vi "Read Data Buffer Subset.vi"(0 "VISA resource name":refnum<visa-resource-name>, 1 "All Data Elements (False)":bool, 2 "Timeout (30000 milliseconds)":u32=30000, 5 "Previous Buffer Read Location (0)":i32, 7 "Next Buffer Location (0)":i32, 9 "Buffer Size (1000)":i32=1000, 11 "error in (no error)":errorcluster) -> (4 "VISA resource name out":refnum<visa-resource-name>, 6 "Measurement Data":dbl[](array[numeric]), 8 "Timestamp":string[](array[string]), 10 "Channel":string[](array[string]), 14 "Reading Number":string[](array[string]), 15 "error out":errorcluster)   [LabVIEW 2020, in "Keithley 27XX.lvlib"]
doc: "It fetches data from the data buffer given the previous buffer location read, and the next buffer location. This VI alone does not initiate a measurement.\n\nNote:\n(1) This VI can be used with continuous initiation to do continuous reads.\n\n(2) Returning all data elements requires ASCII transfers.\n\n(3) Timestamp, Channel, and Reading Number arrays will be left empty if the All Data Elements control is set to False."
uses:
  <instrlib>/Keithley 27XX/Keithley 27XX.lvlib
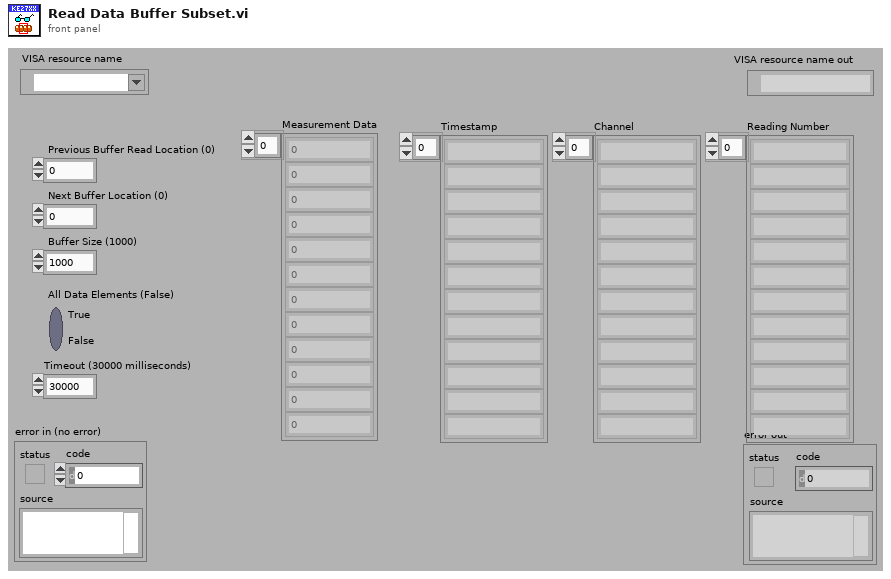
[diagram p1: front panel]
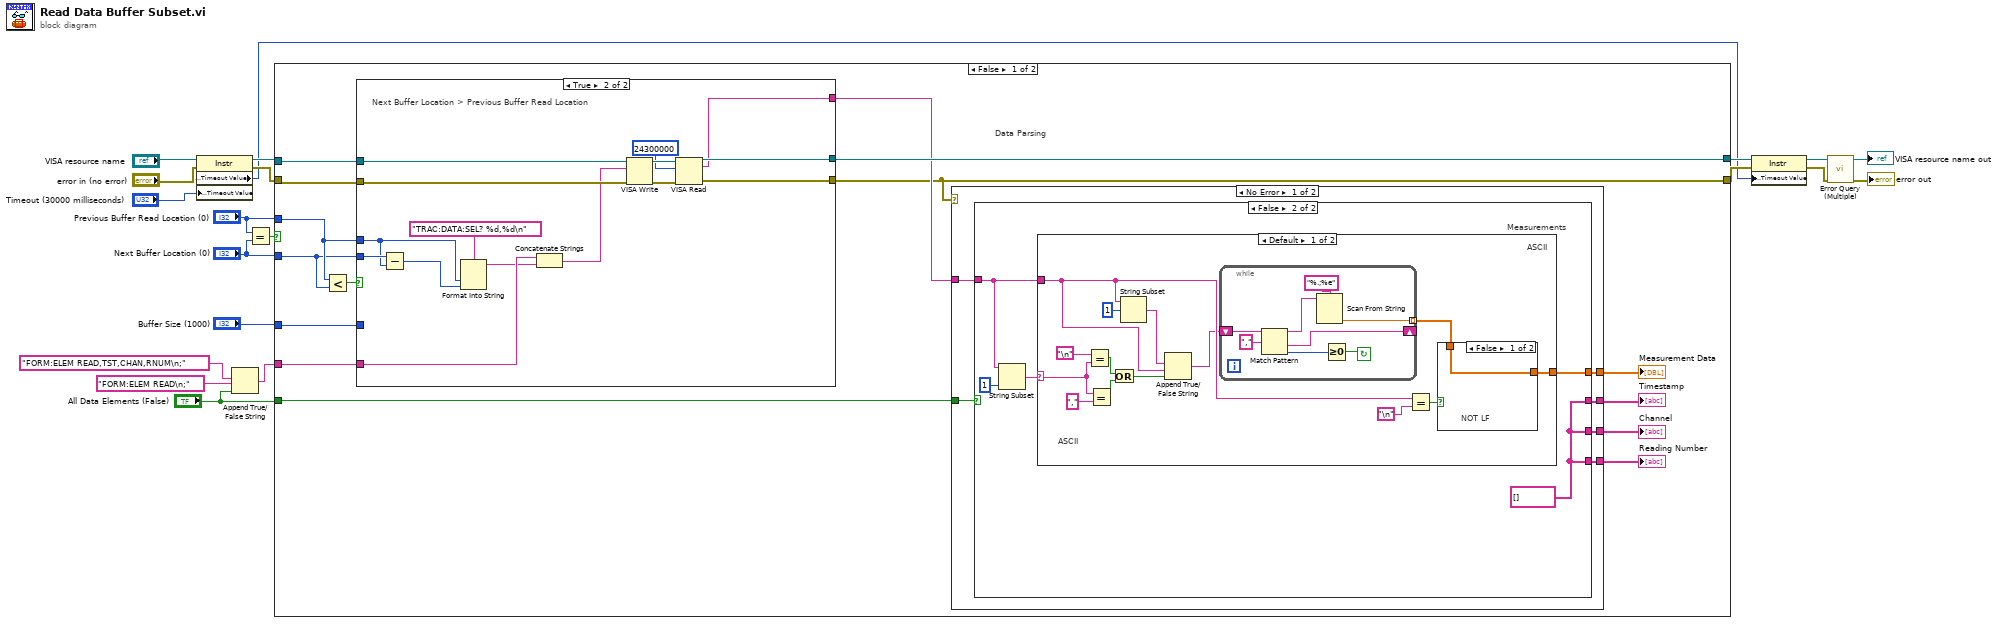
[diagram p0: block diagram]
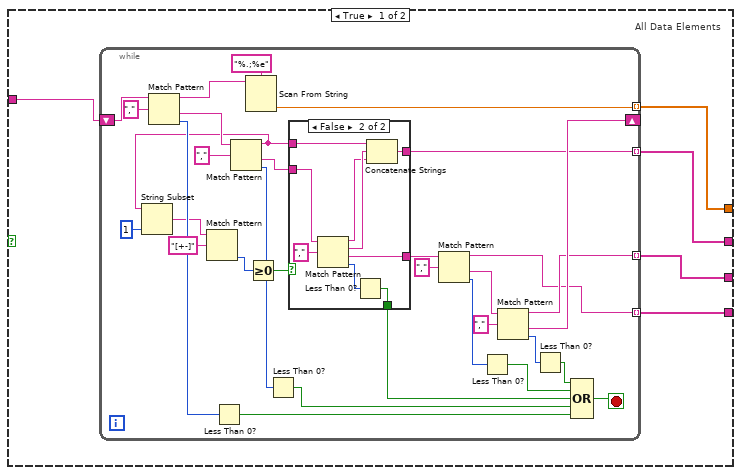
[diagram p2: hidden frame]
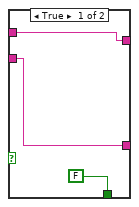
[diagram p3: hidden frame]
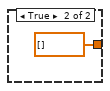
[diagram p4: hidden frame]
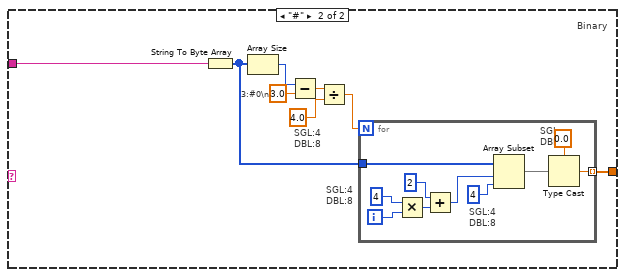
[diagram p5: hidden frame]
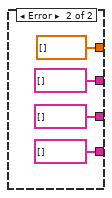
[diagram p6: hidden frame]
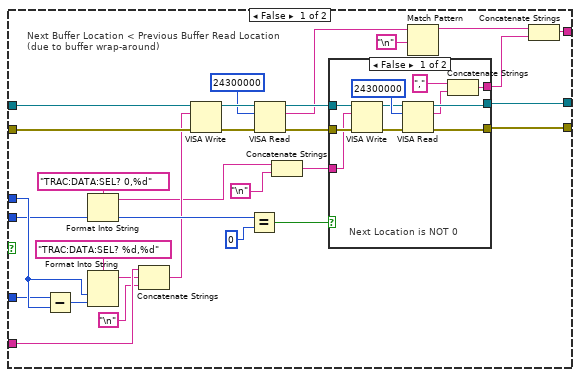
[diagram p7: hidden frame]
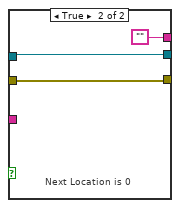
[diagram p8: hidden frame]
diagram:
  n1 = property class="Instr"(reference="VISA resource name", error in="error in (no error)", "General Settings:Timeout Value"="Timeout (30000 milliseconds)") -> (reference out=w12:refnum<visa-resource-name>, error out=w11:errorcluster, "General Settings:Timeout Value"=w6:u32)
  n2 = Append True/False String(1:"All Data Elements (False)", 2:"FORM:ELEM READ\n;" ("false string"), 3:"FORM:ELEM READ,TST,CHAN,RNUM\n;" ("true string")) -> (0:w3:string)  [unwired: 1 in]
  n3 = Equal?(x="Previous Buffer Read Location (0)", y="Next Buffer Location (0)") -> (x = y?=w18:bool)
  n4 = case shown="False" w18 {
    tunnel: "Previous Buffer Read Location (0)" -> [w34 _]
    tunnel: "Next Buffer Location (0)" -> [w27 _]
    tunnel: "Buffer Size (1000)" -> [w33 _]
    tunnel: w12 -> [w30 w201]
    tunnel: w11 -> [w29 w200]
    tunnel: [w31 w201] -> w10
    tunnel: [w21 w200] -> w9
    tunnel: "All Data Elements (False)" -> [w23 _]
    tunnel: w3 -> [w22 _]
    frame False {
      # "Data Parsing"
      n5 = Less?(x=w34, y=w27) -> (x < y?=w35:bool)
      n6 = case shown="True" w35 {
        tunnel: w34 -> [w168 w198]
        tunnel: w27 -> [w159 w199]
        tunnel: w33 -> [w160 _]
        tunnel: [w155 w193] -> w21
        tunnel: [w154 w192] -> w31
        tunnel: w30 -> [w163 w191]
        tunnel: w29 -> [w162 w190]
        tunnel: [w149 w189] -> w28
        tunnel: w22 -> [w170 w187]
        frame False {
          # "Next Buffer Location < Previous Buffer Read Location\n(due to buffer wrap-around)"
          n7 = Subtract(x=w160, y=w168) -> (x-y=w167:i32)
          n8 = Format Into String(format string="TRAC:DATA:SEL? 0,%d", w159) -> (resulting string=w143:string)  [unwired: 2 in, 1 out]
          n9 = Format Into String(format string="TRAC:DATA:SEL? %d,%d", w168, w167) -> (resulting string=w147:string)  [unwired: 2 in, 1 out]
          n10 = Concatenate Strings(w170, w147, "\n") -> (w145:string)
          n11 = VISA Write(VISA resource name=w163, write buffer=w145, error in (no error)=w162) -> (VISA resource name out=w165:refnum<visa-resource-name>, error out=w166:errorcluster)  [unwired: 1 out]
          n12 = Equal?(x=w159, y=0) -> (x = y?=w158:bool)
          n13 = VISA Read(VISA resource name=w165, byte count=u32 24300000, error in (no error)=w166) -> (VISA resource name out=w157:refnum<visa-resource-name>, read buffer=w152:string, error out=w156:errorcluster)  [unwired: 1 out]
          n14 = Concatenate Strings(w143, "\n") -> (w144:string)
          n15 = case shown="False" w158 {
            tunnel: w157 -> [w178 w184]
            tunnel: w156 -> [w177 w183]
            tunnel: [w180 w183] -> w155
            tunnel: [w179 w184] -> w154
            tunnel: w144 -> [w174 _]
            tunnel: [w173 ""] -> w150
            frame False {
              # "Next Location is NOT 0"
              n16 = VISA Write(VISA resource name=w178, write buffer=w174, error in (no error)=w177) -> (VISA resource name out=w175:refnum<visa-resource-name>, error out=w176:errorcluster)  [unwired: 1 out]
              n17 = VISA Read(VISA resource name=w175, byte count=u32 24300000, error in (no error)=w176) -> (VISA resource name out=w179:refnum<visa-resource-name>, read buffer=w172:string, error out=w180:errorcluster)  [unwired: 1 out]
              n18 = Concatenate Strings("," ("y"), w172) -> (w173:string)
            }
            frame True {
              # "Next Location is 0"
            }
          }
          n19 = Match Pattern(string=w152, regular expression="\n") -> (before substring=w151:string)  [unwired: 1 in, 3 out]
          n20 = Concatenate Strings(w151, w150) -> (w149:string)
        }
        frame True {
          # "Next Buffer Location > Previous Buffer Read Location"
          n21 = Subtract(x=w199, y=w198) -> (x-y=w188:i32)
          n22 = Format Into String(format string="TRAC:DATA:SEL? %d,%d\n", w198, w188) -> (resulting string=w186:string)  [unwired: 2 in, 1 out]
          n23 = Concatenate Strings(w187, w186) -> (w185:string)
          n24 = VISA Write(VISA resource name=w191, write buffer=w185, error in (no error)=w190) -> (VISA resource name out=w195:refnum<visa-resource-name>, error out=w196:errorcluster)  [unwired: 1 out]
          n25 = VISA Read(VISA resource name=w195, byte count=u32 24300000, error in (no error)=w196) -> (VISA resource name out=w192:refnum<visa-resource-name>, read buffer=w189:string, error out=w193:errorcluster)  [unwired: 1 out]
        }
      }
      n26 = case shown="No Error" w21 {
        tunnel: [w41 dbl[] []] -> w32
        tunnel: w28 -> [w40 _]
        tunnel: [w39 string[] []] -> w26
        tunnel: [w38 string[] []] -> w25
        tunnel: [w37 string[] []] -> w24
        tunnel: w23 -> [w36 _]
        frame No Error {
          n27 = case shown="False" w36 {
            tunnel: [w45 w95] -> w41
            tunnel: w40 -> [w46 w93]
            tunnel: [w44 w91] -> w39
            tunnel: [w43 w91] -> w38
            tunnel: [w42 w91] -> w37
            frame True {
              # "All Data Elements"
              n28 = while {
                shift-right: [w63] -> _
                shift-left: w46 -> [w74]
                tunnel: [w75] -> w45 mode=indexing
                tunnel: [w55] -> w44 mode=indexing
                tunnel: [w47] -> w42 mode=indexing
                tunnel: [w48] -> w43 mode=indexing
                stop <- w67 stop-if-true
                n29 = Match Pattern(string=w74, regular expression="," ("search string/char (-)")) -> (before substring=w77:string, after substring=w73:string, offset past match=w70:i32)  [unwired: 1 in, 1 out]
                n30 = Less Than 0?(x=w70) -> (x < 0?=w69:bool)
                n31 = Match Pattern(string=w73, regular expression="," ("search string/char (-)")) -> (before substring=w50:string, after substring=w61:string, offset past match=w71:i32)  [unwired: 1 in, 1 out]
                n32 = String Subset(string=w50, length (rest)=1 ("length (rest)")) -> (substring=w51:string)  [unwired: 1 in]
                n33 = Match Pattern(string=w51, regular expression="[+-]") -> (offset past match=w52:i32)  [unwired: 1 in, 3 out]
                n34 = Scan From String(format string="%.;%e", input string=w77) -> (output 1=w75:dbl)  [unwired: 3 in, 3 out]
                n35 = Greater Or Equal To 0?(x=w52) -> (x >= 0?=w53:bool)
                n36 = Less Than 0?(x=w71) -> (x < 0?=w68:bool)
                n37 = case shown="False" w53 {
                  tunnel: [w80 w89] -> w60
                  tunnel: [FALSE w87] -> w56
                  tunnel: w61 -> [w80 w86]
                  tunnel: w50 -> [w79 w85]
                  tunnel: [w79 w82] -> w55
                  frame True {
                  }
                  frame False {
                    n38 = Match Pattern(string=w86, regular expression="," ("search string/char (-)")) -> (before substring=w83:string, match substring=w84:string, after substring=w89:string, offset past match=w88:i32)  [unwired: 1 in]
                    n39 = Less Than 0?(x=w88) -> (x < 0?=w87:bool)
                    n40 = Concatenate Strings(w85, w84, w83) -> (w82:string)
                  }
                }
                n41 = Match Pattern(string=w60, regular expression="," ("search string/char (-)")) -> (before substring=w47:string, after substring=w59:string, offset past match=w58:i32)  [unwired: 1 in, 1 out]
                n42 = Less Than 0?(x=w58) -> (x < 0?=w57:bool)
                n43 = Match Pattern(string=w59, regular expression="," ("search string/char (-)")) -> (before substring=w48:string, after substring=w63:string, offset past match=w66:i32)  [unwired: 1 in, 1 out]
                n44 = Less Than 0?(x=w66) -> (x < 0?=w64:bool)
                n45 = Compound Arithmetic op=OR(w64, w57, w56, w68, w69) -> (w67:bool)
              }
            }
            frame False {
              w91 = string[] []
              # "Measurements"
              n46 = String Subset(string=w93, length (rest)=1 ("length (rest)")) -> (substring=w92:string)  [unwired: 1 in]
              n47 = case shown="Default" w92 {
                selector: w92 -> [w97 _]
                tunnel: w93 -> [w99 w122]
                tunnel: [w108 w120] -> w95
                frame Default {
                  # "ASCII"
                  # "ASCII"
                  n48 = Equal?(x="\n", y=w97) -> (x = y?=w104:bool)
                  n49 = Equal?(x=w97, y=",") -> (x = y?=w103:bool)
                  n50 = Or(x=w104, y=w103) -> (x .or. y?=w101:bool)
                  n51 = String Subset(string=w99, offset (0)=1) -> (substring=w100:string)  [unwired: 1 in]
                  n52 = Append True/False String(1:w101, 2:w99, 3:w100) -> (0:w96:string)  [unwired: 1 in]
                  n53 = while {
                    shift-right: [w113] -> _
                    shift-left: w96 -> [w114]
                    tunnel: [w112] -> w109 mode=indexing
                    stop <- w118 continue-if-true
                    n54 = Match Pattern(string=w114, regular expression="," ("search string/char (-)")) -> (before substring=w117:string, after substring=w113:string, offset past match=w115:i32)  [unwired: 1 in, 1 out]
                    n55 = Scan From String(format string="%.;%e", input string=w117) -> (output 1=w112:dbl)  [unwired: 3 in, 3 out]
                    n56 = Greater Or Equal To 0?(x=w115) -> (x >= 0?=w118:bool)
                  }
                  n57 = Equal?(x=w99, y="\n") -> (x = y?=w106:bool)
                  n58 = case shown="False" w106 {
                    tunnel: w109 -> [w110 _]
                    tunnel: [w110 dbl[] []] -> w108
                    frame False {
                      # "NOT LF"
                    }
                    frame True {
                    }
                  }
                }
                frame "#" {
                  # "Binary"
                  # "3:#0\\n"
                  # "SGL:4\nDBL:8"
                  # "SGL:4\nDBL:8"
                  n59 = String To Byte Array(string=w122) -> (unsigned byte array=w123:u8[])
                  n60 = Array Size(array=w123) -> (size(s)=w127:i32)
                  n61 = Subtract(x=w127, y=3.0) -> (x-y=w124:dbl)
                  n62 = Divide(x=w124, y=4.0) -> (x/y=w121:dbl)
                  n63 = for {
                    N: w121 -> [_]
                    tunnel: w123 -> [w129]
                    tunnel: [w128] -> w120 mode=indexing
                    i -> [w134]
                    # "SGL\nDBL"
                    # "SGL:4\nDBL:8"
                    n64 = Multiply(x=4, y=w134) -> (x*y=w133:i32)
                    n65 = Add(x=2, y=w133) -> (x+y=w130:i32)
                    n66 = Array Subset(array=w129, index=w130, length=4) -> (w136:u8[])
                    n67 = Type Cast(type=sgl 0.0, x=w136) -> (*(type *) &x=w128:sgl)
                  }
                }
              }
            }
          }
        }
        frame Error {
        }
      }
      "Measurement Data" <- w32
      "Timestamp" <- w26
      "Channel" <- w25
      "Reading Number" <- w24
    }
    frame True {
      # "Previous Buffer Read Location = Next Buffer Location\nNo measurements have been taken since the last Read"
    }
  }
  n68 = property class="Instr"(reference=w10, error in=w9, "General Settings:Timeout Value"=w6) -> (reference out=w8:refnum<visa-resource-name>, error out=w7:errorcluster)
  n69 = call <instrlib>:"Error Query (Multiple).vi"("VISA resource name"=w8, "error in (no error)"=w7) -> ("VISA resource name out"=→"VISA resource name out":refnum<visa-resource-name>, "error out"=→"error out":errorcluster)  [unwired: 10 in, 2 out]
